vi "midiInEventsToReceive.vi"(8 "error in":errorcluster, 10 "Event Array":u8[](array[numeric]), 11 "midi in":refnum<class "midi.lvclass">) -> (0 "error out":errorcluster, 3 "midi out":refnum<class "midi.lvclass">)   [LabVIEW 2020, in "midi.lvclass"]
doc: "The midiInClose function closes the specified MIDI input device."
uses:
  midi.lvclass
  midi.lvclass/midi.ctl
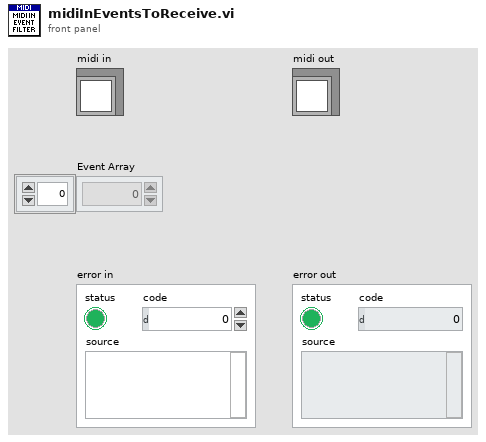
[diagram p1: front panel]
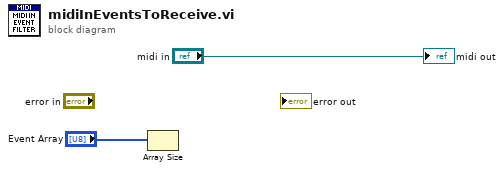
[diagram p0: block diagram]
diagram:
  n1 = Array Size(array="Event Array") -> ()  [unwired: 1 out]
  "midi out" <- "midi in"
